vi "Example 1 Event.vi"() -> ()   [LabVIEW 2015]
panel:
  in  "Reset (T)":bool
  out "error out":errorcluster
  in  "Language Selector":i16(ring)=1 items=["GEN", "SCPI"]
  in  "Address":i16=6
  in  "Baud Rate":i32(ring)=6 items=["1200", "2400", "4800", "9600", "19200", "38400", "57600", "115200"]
  in  "error in":errorcluster
  in  "VISA":refnum<visa-resource-name>
  in  "y":bool
  out "Output Power":dbl format="%.4f"
  out "Output Current":dbl format="%.4f"
  out "Output Voltage":dbl format="%.4f"
  in  "Output ON":bool=TRUE
  in  "Voltage Limit":dbl format="%.4f"
  in  "Current Limit":dbl=3.0 format="%.4f"
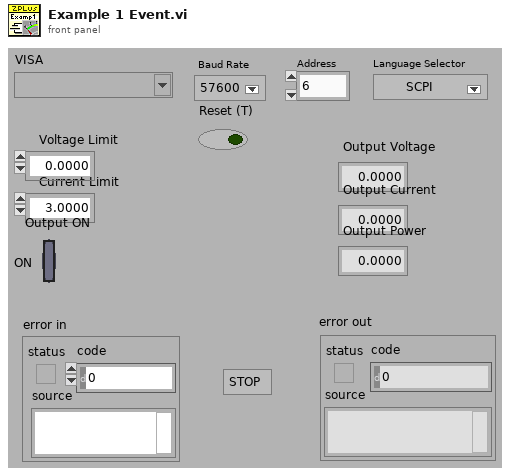
[diagram p1: front panel]
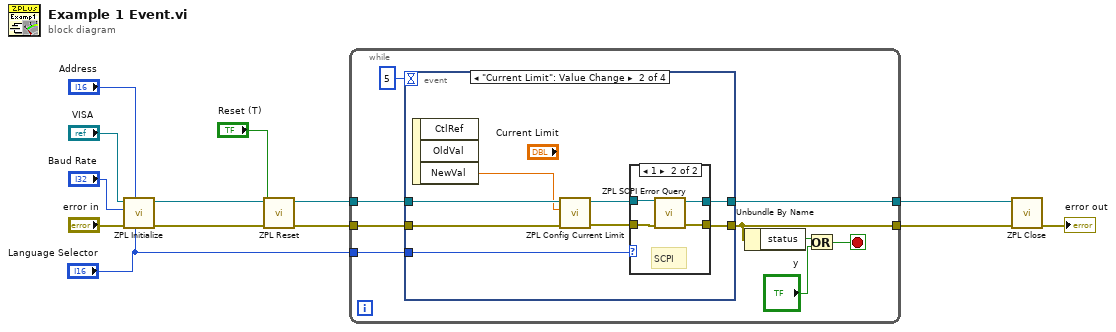
[diagram p0: block diagram]
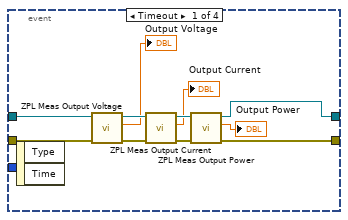
[diagram p2: hidden frame]
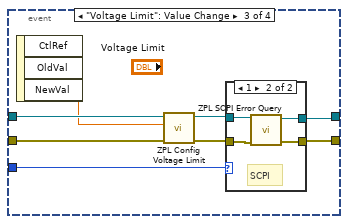
[diagram p4: hidden frame]
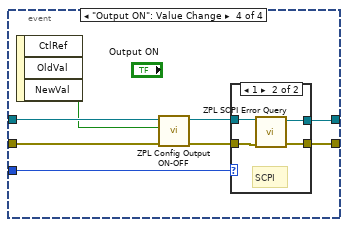
[diagram p6: hidden frame]
diagram:
  n1 = call "ZPL Initialize.vi"("Language Selector"="Language Selector", "Address"="Address", "error in"="error in", "Baud Rate"="Baud Rate", "VISA"="VISA") -> ("error out"=w3:errorcluster, "VISA  out"=w2:refnum<visa-resource-name>)  [unwired: 3 in, 2 out]
  n2 = call "ZPL Reset.vi"("error"=w3, "Reset (T)"="Reset (T)", "VISA"=w2) -> ("error out"=w5:errorcluster, "VISA out"=w6:refnum<visa-resource-name>)  [unwired: 7 in]
  n3 = while {
    tunnel: w6 -> [w22]
    tunnel: [w16] -> w13
    tunnel: w5 -> [w21]
    tunnel: [w15] -> w12
    tunnel: "Language Selector" -> [w14]
    stop <- w19 stop-if-true
    n4 = event shown="[1] \"Current Limit\": Value Change" {
      selector: _ -> [_ _ _ _]
      dyn-events: _ -> [_ _ _ _]
      timeout: 5 -> [_ _ _ _]
      tunnel: w22 -> [w33 w41 w55 w69]
      tunnel: [w27 w36 w50 w63] -> w16
      tunnel: w21 -> [w30 w40 w54 w68]
      tunnel: [w28 w35 w49 w62] -> w15
      tunnel: w14 -> [_ w34 w48 w66]
      event Timeout {
        n5 = event-data() -> ()  [unwired: 1 in, 2 out]
        n6 = call "ZPL Meas Output Voltage.vi"("error"=w30, "VISA"=w33) -> ("error out"=w23:errorcluster, "Output Voltage"=→"Output Voltage":dbl, "VISA out"=w32:refnum<visa-resource-name>)  [unwired: 7 in]
        n7 = call "ZPL Meas Output Current.vi"("error"=w23, "VISA"=w32) -> ("error out"=w29:errorcluster, "Output Current"=→"Output Current":dbl, "VISA out"=w31:refnum<visa-resource-name>)  [unwired: 7 in]
        n8 = call "ZPL Meas Output Power.vi"("error"=w29, "VISA"=w31) -> ("error out"=w28:errorcluster, "Output Power"=→"Output Power":dbl, "VISA out"=w27:refnum<visa-resource-name>)  [unwired: 7 in]
      }
      event "Current Limit": Value Change {
        n9 = event-data() -> ("NewVal"=w39:dbl)  [unwired: 1 in, 2 out]
        n10 = call "ZPL Config Current Limit.vi"("error"=w40, "Current Limit"=w39, "VISA"=w41) -> ("error out"=w37:errorcluster, "VISA out"=w38:refnum<visa-resource-name>)  [unwired: 7 in]
        n11 = case shown="1" w34 {
          tunnel: w38 -> [w43 w47]
          tunnel: w37 -> [w42 w46]
          tunnel: [w43 w45] -> w36
          tunnel: [w42 w44] -> w35
          frame 0, Default {
            # "GEN"
          }
          frame 1 {
            # "SCPI"
            n12 = call "ZPL SCPI Error Query.vi"("error"=w46, "VISA"=w47) -> ("error out"=w44:errorcluster, "VISA out"=w45:refnum<visa-resource-name>)  [unwired: 6 in, 2 out]
          }
        }
      }
      event "Voltage Limit": Value Change {
        n13 = event-data() -> ("NewVal"=w53:dbl)  [unwired: 1 in, 2 out]
        n14 = call "ZPL Config Voltage Limit.vi"("error"=w54, "Voltage Limit"=w53, "VISA"=w55) -> ("error out"=w51:errorcluster, "VISA out"=w52:refnum<visa-resource-name>)  [unwired: 7 in]
        n15 = case shown="1" w48 {
          tunnel: w52 -> [w57 w61]
          tunnel: w51 -> [w56 w60]
          tunnel: [w57 w59] -> w50
          tunnel: [w56 w58] -> w49
          frame 0, Default {
            # "GEN"
          }
          frame 1 {
            # "SCPI"
            n16 = call "ZPL SCPI Error Query.vi"("error"=w60, "VISA"=w61) -> ("error out"=w58:errorcluster, "VISA out"=w59:refnum<visa-resource-name>)  [unwired: 6 in, 2 out]
          }
        }
      }
      event "Output ON": Value Change {
        n17 = event-data() -> ("NewVal"=w67:bool)  [unwired: 1 in, 2 out]
        n18 = call "ZPL Config Output ON-OFF.vi"("error"=w68, "Output ON"=w67, "VISA"=w69) -> ("error out"=w64:errorcluster, "VISA out"=w65:refnum<visa-resource-name>)  [unwired: 7 in]
        n19 = case shown="1" w66 {
          tunnel: w65 -> [w71 w75]
          tunnel: w64 -> [w70 w74]
          tunnel: [w71 w73] -> w63
          tunnel: [w70 w72] -> w62
          frame 0, Default {
            # "GEN"
          }
          frame 1 {
            # "SCPI"
            n20 = call "ZPL SCPI Error Query.vi"("error"=w74, "VISA"=w75) -> ("error out"=w72:errorcluster, "VISA out"=w73:refnum<visa-resource-name>)  [unwired: 6 in, 2 out]
          }
        }
      }
    }
    n21 = Unbundle By Name(w15) -> ("status"=w18:bool)
    n22 = Or(x=w18, y="y") -> (x .or. y?=w19:bool)
  }
  n23 = call "ZPL Close.vi"("error"=w12, "VISA name"=w13) -> ("error out"=→"error out":errorcluster)  [unwired: 7 in]
